vi "RefreshTestTreeScript.vi"(8 "error in (no error)":errorcluster, 11 "TestListboxRef":refnum<vi>) -> (0 "error out":errorcluster, 3 "String":string)   [LabVIEW 2018]
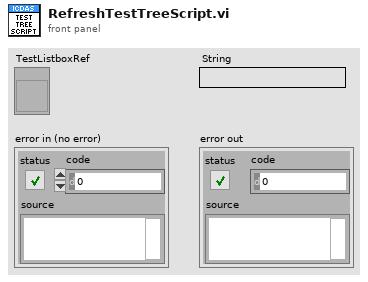
[diagram p1: front panel]
types:
  T1 = typedef "Plugin Tree Tag.ctl" = cluster{"ItemType":T2, "Name":string, "Path":path, "Script":string[]}
  T2 = typedef "Plugins Tree Item Type.ctl" = enum16{"Plugin", "Instrument", "INI File", "INI Script"}
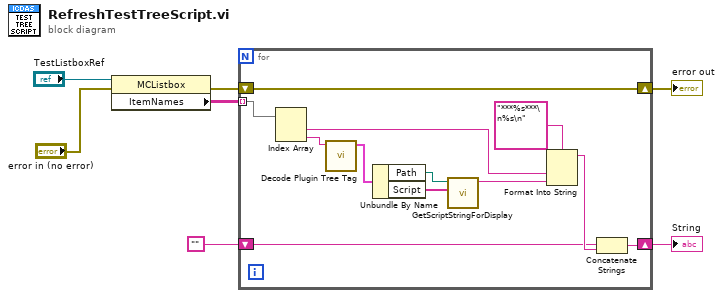
[diagram p0: block diagram]
diagram:
  n1 = property class="MCListbox"(reference="TestListboxRef", error in="error in (no error)") -> (error out=w3:errorcluster, "ItemNames"=w2:string[][])  [unwired: 1 out]
  n2 = for {
    tunnel: w2 -> [w11] mode=indexing
    shift-right: [w18] -> w7
    shift-left: w3 -> [w18]
    shift-right: [w15] -> w5
    shift-left: "" -> [w14]
    n3 = Index Array(array=w11) -> (element #1=w10:string, element #2=w9:string)  [unwired: 2 in]
    n4 = call "Decode Plugin Tree Tag.vi"("Tag"=w9) -> ("Plugin Tree Tag"=w19:T1)  [unwired: 9 in, 1 out]
    n5 = Unbundle By Name(w19) -> ("Path"=w8:path, "Script"=w13:string[])
    n6 = call "GetScriptStringForDisplay.vi"("Script"=w13, "INI File Path"=w8) -> ("Script String"=w12:string)  [unwired: 9 in]
    n7 = Format Into String(format string="***%s***\n%s\n", w10, w12) -> (resulting string=w16:string)  [unwired: 2 in, 1 out]
    n8 = Concatenate Strings(w14, w16) -> (w15:string)
  }
  "error out" <- w7
  "String" <- w5
